vi "Example.vi"() -> ()   [LabVIEW 2015, in "CnPt.lvclass"]
uses:
  CnPt.lvclass
  <vilib>/MSR Consulting, LLC/General Reuse/Session APIs/File Access/Config Data/Config Data.lvclass
  <vilib>/MSR Consulting, LLC/General Reuse/Session APIs/File Access/Config Data/Config Session.ctl
  <vilib>/Platform/TimedLoop/XDataNode/timing_clust.ctl
  <vilib>/Platform/TimedLoop/XDataNode/nitl_modes.ctl
  <vilib>/Platform/TimedLoop/XDataNode/wakeup.ctl
  <vilib>/MSR Consulting, LLC/General Reuse/Session APIs/File Access/Config Data/Config Data.lvclass/Config Data.ctl
  <vilib>/MSR Consulting, LLC/Devices/Configurable Device/Configurable Device.lvclass/Configurable Device.ctl
  CnPt.lvclass/CnPt.ctl
  <vilib>/MSR Consulting, LLC/General Reuse/Data/Double/Double.lvclass
  <vilib>/MSR Consulting, LLC/General Reuse/Session APIs/File Access/Config Data/Accessors/Write Cfg Path.vi
  <vilib>/MSR Consulting, LLC/Devices/Configurable Device/Write Handle.vi
  Accessors/Read Tsp.vi
  <vilib>/Platform/TimedLoop/XDataNode/XDataNode.xnode
  <vilib>/MSR Consulting, LLC/General Reuse/Session APIs/_Session Fwk/Session - Root.lvclass
  <vilib>/Platform/TimedLoop/XDataNode/XDNodeRunTimeDep.lvlib
panel:
  out "error out":errorcluster
  in  "Tsp":dbl
  out "temperature":dbl(graph)
  out "Config directory":path
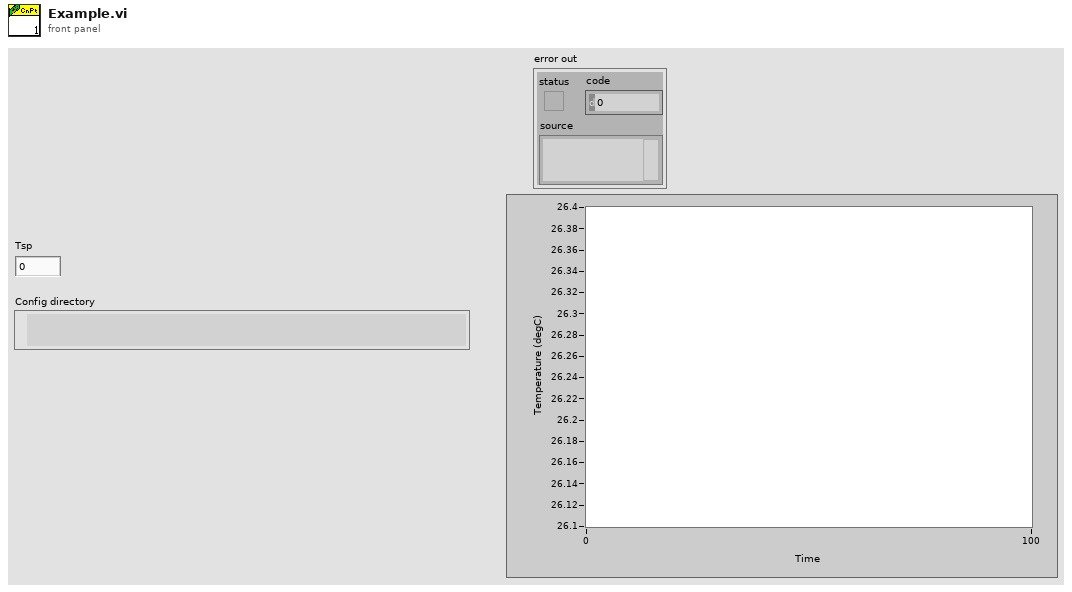
[diagram p1: front panel]
types:
  T1 = typedef "Config Data.lvclass/Config Session.ctl" = refnum<data-value>
  T2 = typedef "Session - Root.lvclass/Session Handle.ctl" = refnum<data-value>
  T3 = typedef "XDNodeRunTimeDep.lvlib/timing_clust.ctl" = cluster{"Expected End [f-1]":u64, "Actual End [f-1]":u64, "Finished Late? [f-1]":bool, "Expected End [i-1]":u64, "Actual End [i-1]":u64, "Finished Late? [i-1]":bool, "Expected Start [i]":u64, "Actual Start [i]":u64, "Expected Start [f]":u64, "Actual Start [f]":u64, "Source Name":string, "Structure Name":string, "Period":i64, "Deadline":i64, "Offset":i64, "Start":i64, "Priority":i32, "Timeout":i32, "Mode":T4, "Wakeup Reason":T5, "Error":errorcluster, "Source Type":string, "Secondary Source Type":string, "Global End Time":u64, "Global Start Time":u64, "Frame Duration":u64, "Iteration Duration":u64, "Assigned CPU":i32, "I/O Scan Engine Mode":u32}
  T4 = typedef "XDNodeRunTimeDep.lvlib/nitl_modes.ctl" = enum32{"No Change", "Process missed periods, maintain original phase", "Discard missed periods, maintain original phase", "Process missed periods, ignore original phase", "Discard missed periods, ignore original phase"}
  T5 = typedef "XDNodeRunTimeDep.lvlib/wakeup.ctl" = enum32{"Normal", "Aborted", "Asynchronous wakeup", "Timing source error", "Timed loop error", "Timeout"}
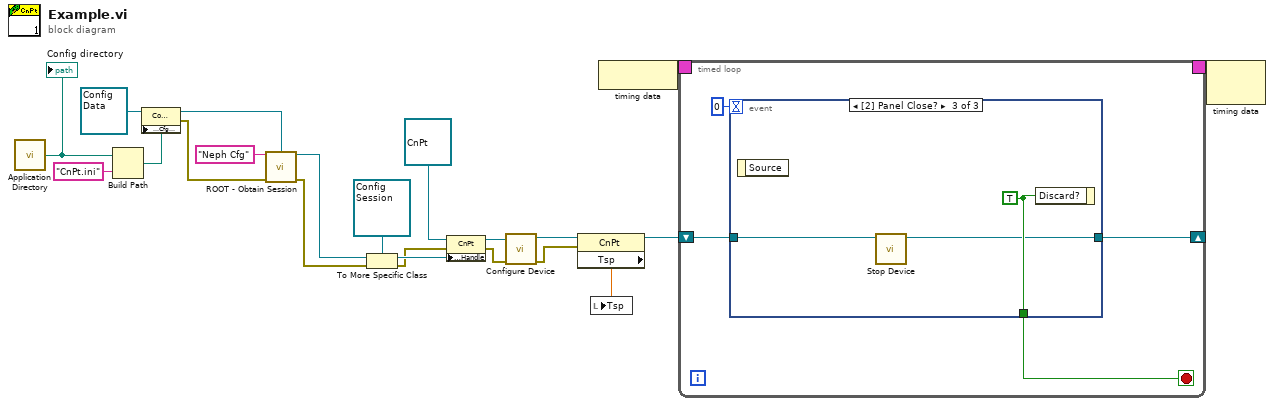
[diagram p0: block diagram]
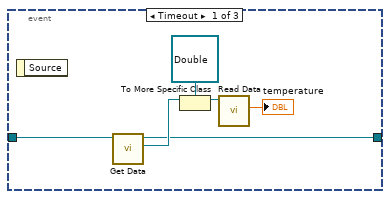
[diagram p2: hidden frame]
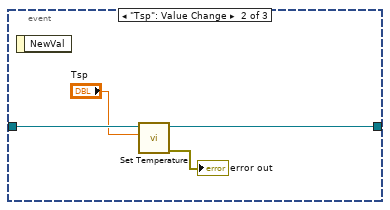
[diagram p3: hidden frame]
diagram:
  n1 = call <vilib>:"Application Directory.vi"() -> ("Application Directory"=w11:path)
  "Config directory" <- w11
  n2 = Build Path(base path=w11, name or relative path="CnPt.ini") -> (appended path=w12:path)
  n3 = property class="Config Data"(reference=refnum<class "Config Data.lvclass"> refnum ("Config Data"), "Accessors:Cfg Path"=w12) -> (reference out=w20:refnum<class "Config Data.lvclass">, error out=w5:errorcluster)  [unwired: 1 in]
  n4 = call <vilib>:"ROOT - Obtain Session.vi"("Session Name ()"="Neph Cfg", "OBJ - Session"=w20, "error in (no error)"=w5) -> ("Session Handle"=w17:T2, "error out"=w14:errorcluster)  [unwired: 10 in, 1 out]
  n5 = To More Specific Class(target class=T1 refnum ("Session Handle"), reference=w17, error in=w14) -> (specific class reference=w16:T1, error out=w15:errorcluster)
  n6 = property class="CnPt"(reference=refnum<class "CnPt.lvclass"> refnum ("CnPt"), error in=w15, "Accessors:Handle"=w16) -> (reference out=w9:refnum<class "CnPt.lvclass">, error out=w8:errorcluster)
  n7 = call-dynamic "Configure Device.vi"("error in"=w8, "CnPt in"=w9) -> ("error out"=w1:errorcluster, "CnPt out"=w4:refnum<class "CnPt.lvclass">)  [unwired: 6 in, 2 out]
  n8 = property class="CnPt"(reference=w4, error in=w1) -> (reference out=w3:refnum<class "CnPt.lvclass">, "Tsp"=w2:dbl)  [unwired: 1 out]
  n9 = local write "Tsp"(w2) -> ()
  n10 = node-c288() -> (w7:T3)
  n11 = timed-loop {
    timing: w7 -> [_]
    timing-out: [_] -> w6
    shift-right: [w22] -> _
    shift-left: w3 -> [w24]
    stop <- w23 stop-if-true
    n12 = event shown="[2] Panel Close?" {
      selector: _ -> [_ _ _]
      dyn-events: _ -> [_ _ _]
      timeout: 0 -> [_ _ _]
      tunnel: w24 -> [w31 w35 w37]
      tunnel: [_ _ w38] -> w23
      tunnel: [w26 w32 w36] -> w22
      event Timeout {
        n13 = event-data() -> ()  [unwired: 1 in, 1 out]
        n14 = call-dynamic "Get Data.vi"("Cfg Dev in"=w31) -> ("Data"=w30:refnum<class "Data.lvclass">, "Cfg Dev out"=w26:refnum<class "CnPt.lvclass">)  [unwired: 8 in, 1 out]
        n15 = To More Specific Class(target class=refnum<class "Double.lvclass"> refnum ("Base Data Lib:Double"), reference=w30) -> (specific class reference=w29:refnum<class "Double.lvclass">)  [unwired: 1 in, 1 out]
        n16 = call <vilib>:"Read Data.vi"("Double in"=w29) -> ("Data"=→"temperature":dbl)  [unwired: 8 in, 2 out]
      }
      event "Tsp": Value Change {
        n17 = event-data() -> ()  [unwired: 1 in, 1 out]
        n18 = call "Set Temperature.vi"("Temperature"="Tsp", "CnPt in"=w35) -> ("error out"=→"error out":errorcluster, "CnPt out"=w32:refnum<class "CnPt.lvclass">)  [unwired: 8 in]
      }
      event Panel Close? {
        w38 = TRUE ("Discard?")
        n19 = event-data() -> ()  [unwired: 1 in, 1 out]
        n20 = call-dynamic "Stop Device.vi"("CnPt in"=w37) -> ("CnPt out"=w36:refnum<class "CnPt.lvclass">)  [unwired: 9 in, 1 out]
        n21 = event-data("Discard?"=w38) -> ()  [unwired: 1 in, 1 out]
      }
    }
  }
  n22 = node-c288(w6) -> ()  [unwired: 1 out]
